vi "Set Glow Plug Duty Cycle.vi"(8 "Error In":errorcluster, 10 "Duty Cycle":i32, 11 "ECU COM Port":refnum<visa-resource-name>) -> (0 "Error Out":errorcluster, 3 "ECU COM Port Out":refnum<visa-resource-name>)   [LabVIEW 2017]
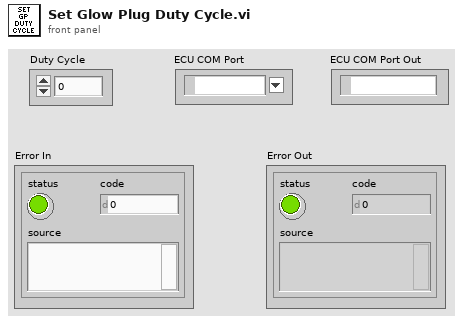
[diagram p1: front panel]
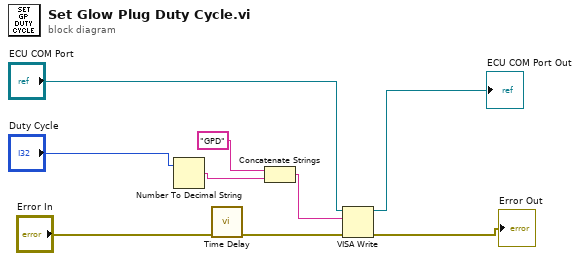
[diagram p0: block diagram]
diagram:
  n1 = Number To Decimal String(number="Duty Cycle") -> (decimal integer string=w8:string)  [unwired: 1 in]
  n2 = call "Time Delay"("error in (no error)"="Error In") -> ("error out"=w1:errorcluster)  [unwired: 10 in]
  n3 = Concatenate Strings("GPD" ("write buffer"), w8) -> (w9:string)
  n4 = VISA Write(VISA resource name="ECU COM Port", write buffer=w9, error in (no error)=w1) -> (VISA resource name out=→"ECU COM Port Out":refnum<visa-resource-name>, error out=→"Error Out":errorcluster)  [unwired: 1 out]
